vi "索引数组函数.vi"() -> ()   [LabVIEW 2014]
panel:
  out "子数组":dbl[](array[numeric])
  out "元素":dbl
  out "二维数组":dbl[][](array[numeric])
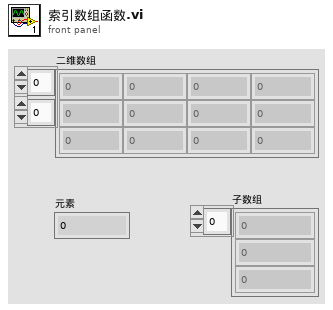
[diagram p1: front panel]
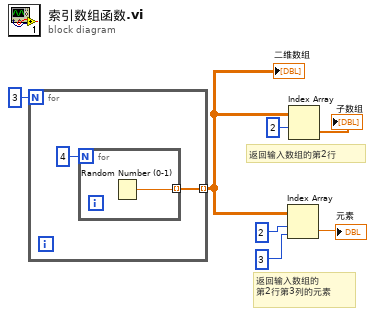
[diagram p0: block diagram]
diagram:
  # "返回输入数组的第2行"
  # "返回输入数组的\n第2行第3列的元素"
  n1 = for {
    N: 3 -> [_]
    tunnel: [w8] -> w3 mode=indexing
    n2 = for {
      N: 4 -> [_]
      tunnel: [w10] -> w8 mode=indexing
      n3 = Random Number (0-1)() -> (number: 0 to 1=w10:dbl)
    }
  }
  "二维数组" <- w3
  n4 = Index Array(array=w3, index (row)=2 ("索引 (行)"), index (col)=3 ("禁用的索引 (列)")) -> (element=→"元素":dbl)
  n5 = Index Array(array=w3, index (row)=2 ("索引 (行)")) -> (element=→"子数组":dbl[])  [unwired: 1 in]
